vi "Read TDMS File.vi"(8 "Error In":errorcluster, 9 "Channel":string="TDO", 11 "File Path Control":path=path "\\\\eden\\NHMFLDATA/Data/cell3daq/January_2020/012820/p012_012820.tdms") -> (0 "Error Out":errorcluster, 1 "Waveform":waveform(dbl), 3 "File out":path=path "\\\\eden\\NHMFLDATA/Data/cell3daq/January_2020/012820/p012_012820.tdms")   [LabVIEW 2019]
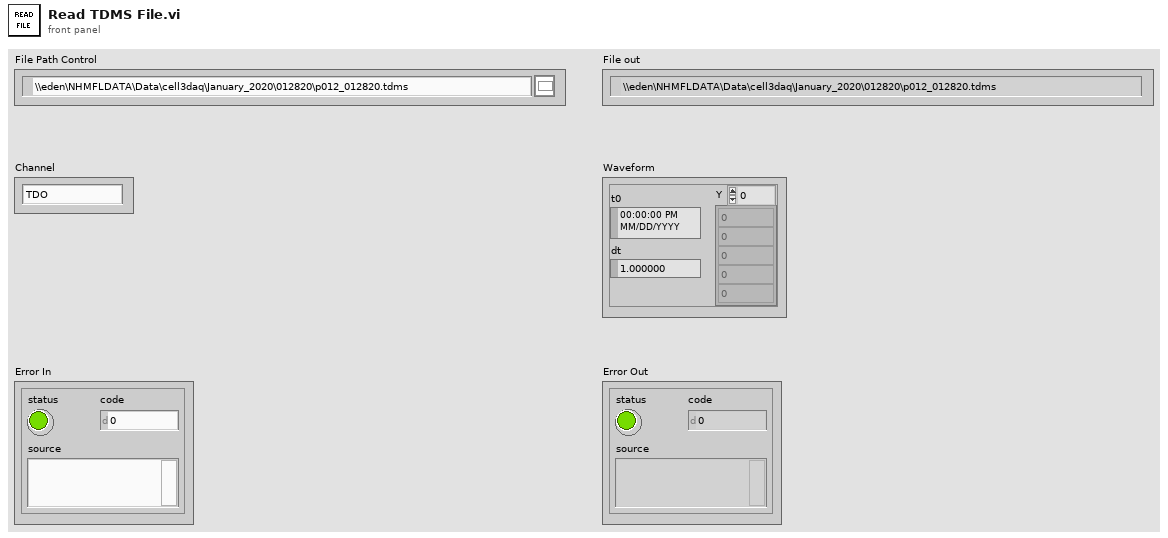
[diagram p1: front panel]
types:
  T1 = enum16{"open", "open or create", "create or replace", "create", "open (read-only)"}
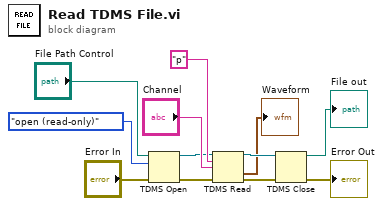
[diagram p0: block diagram]
diagram:
  n1 = TDMS Open(8:"Error In", 10:T1."open (read-only)" ("operation (0:open)"), 11:"File Path Control") -> (0:w8:errorcluster, 3:w9:refnum<k34>)  [unwired: 4 in]
  n2 = TDMS Read(0:w9, 5:"p" ("group name in"), 7:"Channel", 11:w8) -> (4:w7:refnum<k34>, 10:→"Waveform":waveform(dbl), 15:w6:errorcluster)  [unwired: 4 in, 3 out]
  n3 = TDMS Close(8:w6, 11:w7) -> (0:→"Error Out":errorcluster, 3:→"File out":path)
